vi "TemplateGUITAF_ClassCast.vi"(11 "TemplateGUITAF in":refnum<class>) -> (3 "TemplateGUITAF out":refnum<class "TemplateGUITAF.lvclass">)   [LabVIEW 2021, in "TemplateGUITAF.lvlib" / "TemplateGUITAF.lvclass"]
uses:
  TemplateGUITAF.lvclass
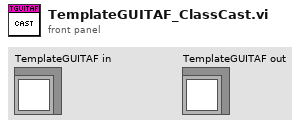
[diagram p1: front panel]
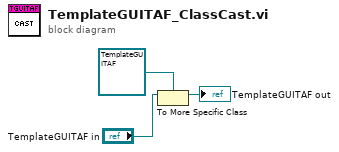
[diagram p0: block diagram]
diagram:
  n1 = To More Specific Class(target class=refnum<class "TemplateGUITAF.lvclass"> refnum ("reference in"), reference="TemplateGUITAF in") -> (specific class reference=→"TemplateGUITAF out":refnum<class "TemplateGUITAF.lvclass">)  [unwired: 1 in, 1 out]
